vi "SS_acquire_data.vi"(0 "Type":refnum<k20>, 1 "idx":i32, 5 "SweptSines (in)":T3={"Log-Channel_select"=[FALSE, FALSE, FALSE, FALSE, FALSE, FALSE], "JSON Header"="", "SS-Params-Array"=[], "input_frequency_definitions"={"Amp"=0.0, "Ts"=0.0, "num_periodsMT"=[], "freqs_Hz"=[], "numAve_s"=[], "Nsamp_total"=[], "Nsettle_s"=[], "Ncollect_s"=[]}, "DAC-ADC primary 2"=0, "Channel-Names"=[], "num_chan"=0, "num-freqs"=0, "Input File (json)"=path "Z:/mpc-journal/sysID/FRF_data/x-axis_sines_info.json"} {"DAC-ADC primary 2" items=["DAC0/ADC0", "DAC1/ADC1", "DAC2/ADC2", "DAC3/ADC3", ""]}, 11 "error in":errorcluster, 12 "Signal Amplitude (V)":dbl=1.0) -> (4 "FPGA Interface out":T6, 6 "SweptSines (out)":T3={"Log-Channel_select"=[FALSE, FALSE, FALSE, FALSE, FALSE, FALSE], "JSON Header"="", "SS-Params-Array"=[], "input_frequency_definitions"={"Amp"=0.0, "Ts"=0.0, "num_periodsMT"=[], "freqs_Hz"=[], "numAve_s"=[], "Nsamp_total"=[], "Nsettle_s"=[], "Ncollect_s"=[]}, "DAC-ADC primary 2"=0, "Channel-Names"=[], "num_chan"=0, "num-freqs"=0, "Input File (json)"=path "Z:/mpc-journal/sysID/FRF_data/x-axis_sines_info.json"} {"DAC-ADC primary 2" items=["DAC0/ADC0", "DAC1/ADC1", "DAC2/ADC2", "DAC3/ADC3", ""]}, 10 "experiment-data":T1, 15 "error IO":errorcluster)   [LabVIEW 2017]
uses:
  controls/SS_fpga_sysID_REFTYPE.ctl
  controls/SS_SweptSines.ctl
  controls/SS_sin_params.ctl
  controls/SS_input_data_json.ctl
  controls/SS_experimental-data.ctl
  controls/SS_FourierData.ctl
  fpga_interface_lib/fpga_interface_types/fpga-swept-sines-dynamic-ref.ctl
  <vilib>/Utility/error.llb/DialogType.ctl
  <vilib>/Utility/error.llb/Error Cluster From Error Code.vi
  <vilib>/rvi/errors/niLvFpgaAdjustHostInterfaceError.vi
  fpga_interface_lib/acquire_FXP_16-5_FIFO_1.vi
  <vilib>/rvi/interface/nirviReadWriteControl/nirviReadWriteControl.xnode
  c-src/sweptSines_lib/libsweptsines.dll
  fpga_interface_lib/fpga_interface.lvlib
  <vilib>/rvi/interface/Simulation/niFpgaSimulationCallBeginRW.vi
  NiFpgaLv.dll
panel:
  out "Type out":refnum<k20>
  in  "experiment-data--":T1
  in  "DDS_params":T7={"Accumulator Increment"=100000, "Phase Shift"=0, "Signal Amplitude (x 2^15)"=32768}
  out "iter":i32
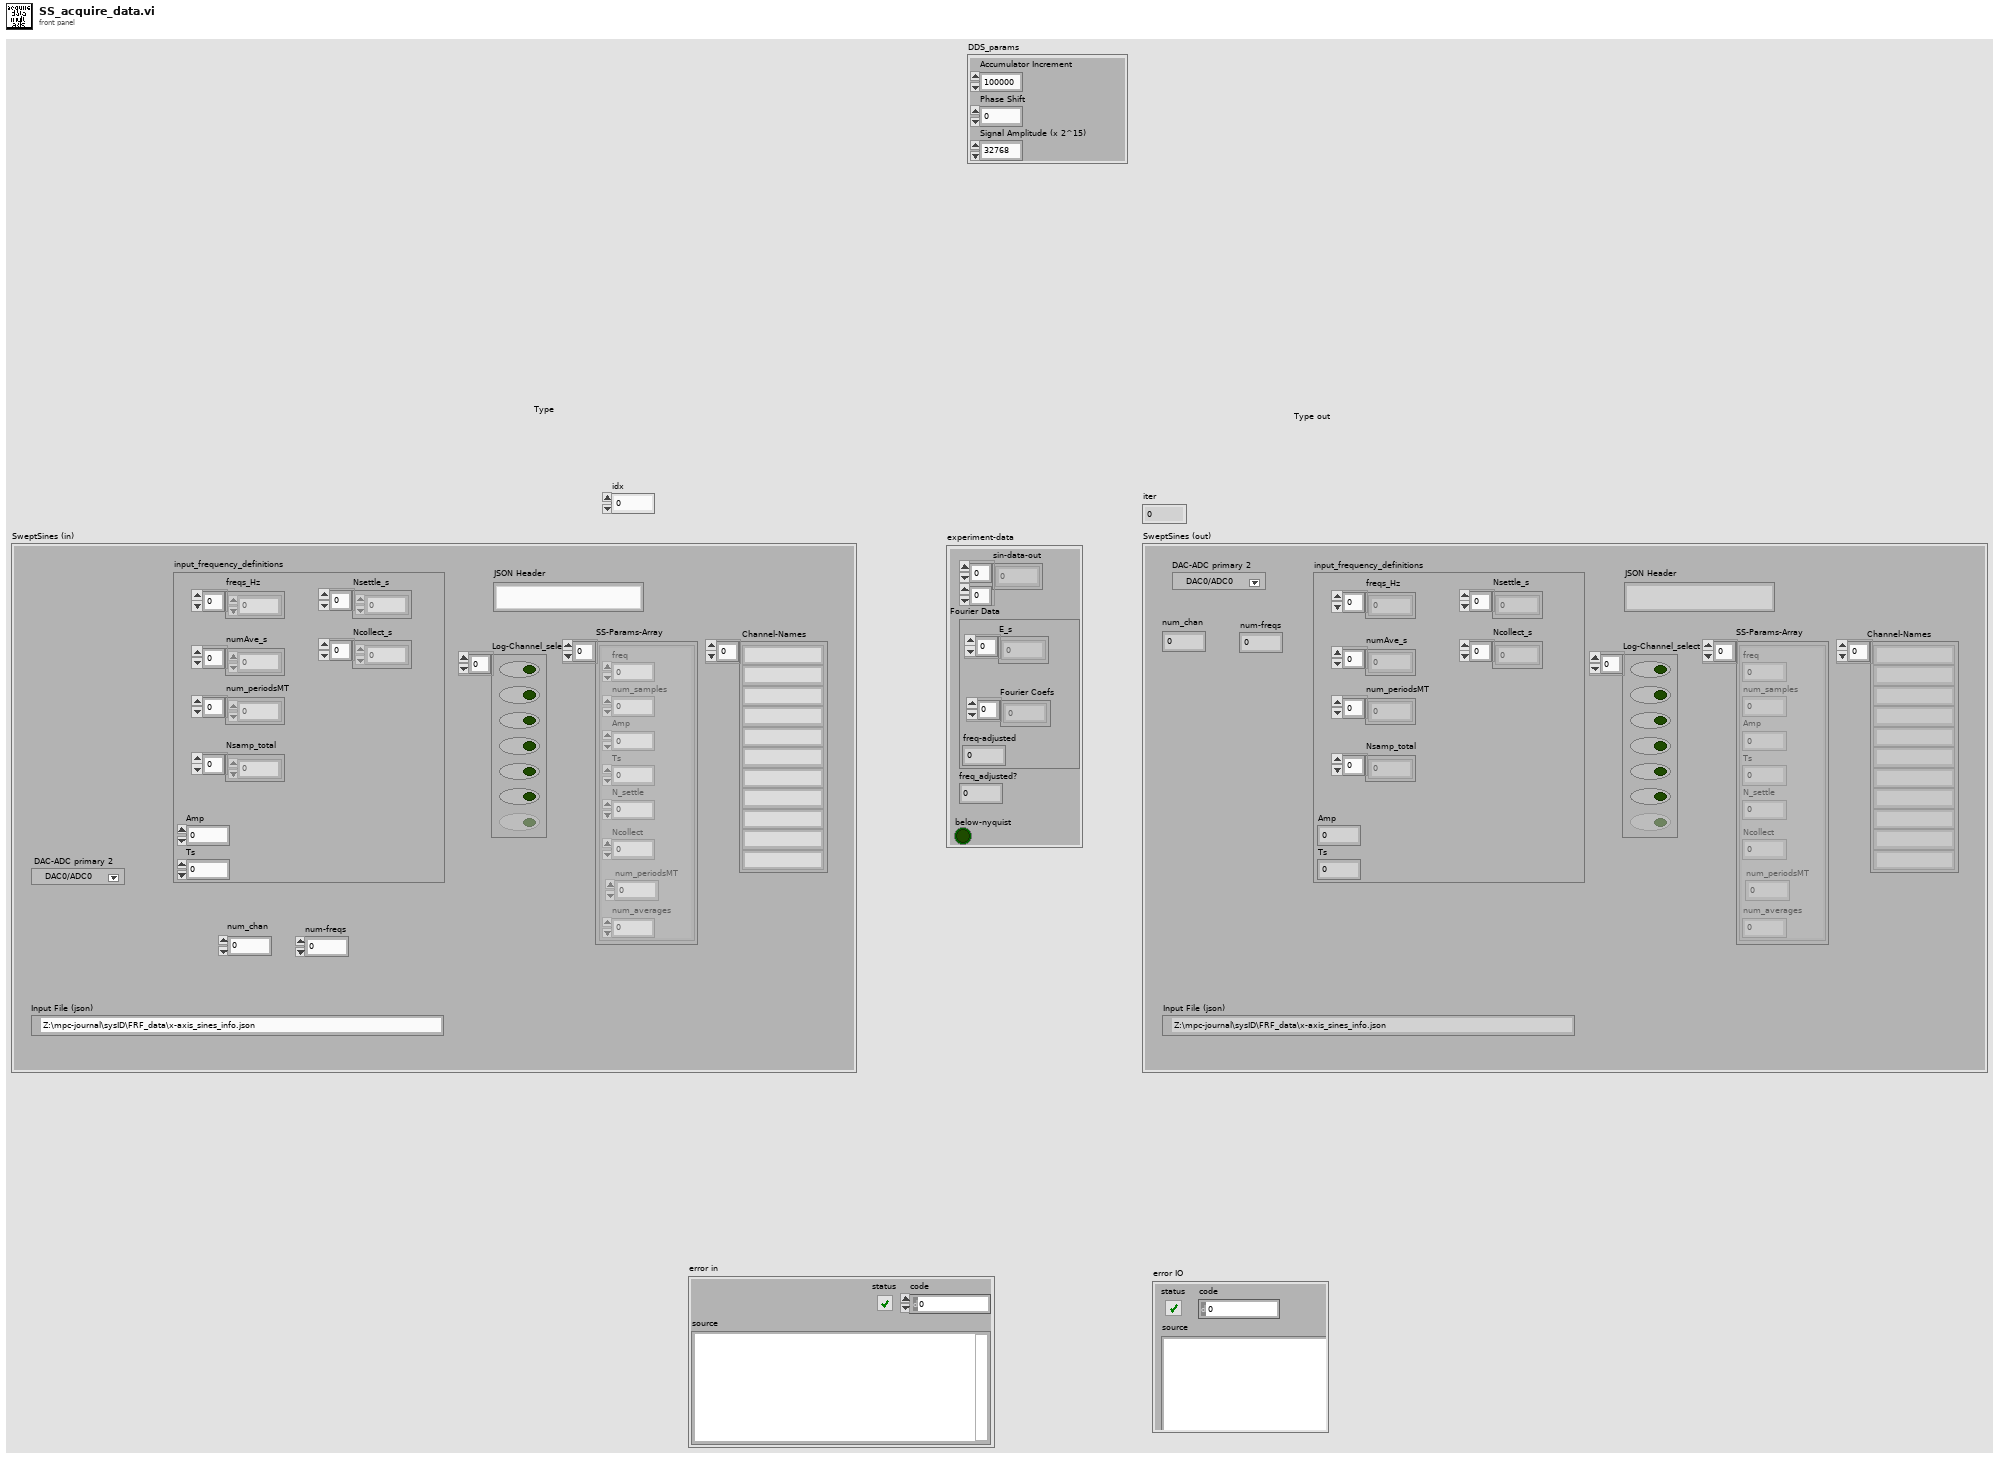
[diagram p1: front panel]
types:
  T1 = typedef "SS_experimental-data.ctl" = cluster{"sin-data-out":dbl[][], "Fourier Data":T2, "freq_adjusted?":dbl, "below-nyquist":bool}
  T2 = typedef "SS_FourierData.ctl" = cluster{"E_s":dbl[], "Fourier Coefs":cdb[], "freq-adjusted":dbl}
  T3 = typedef "SS_SweptSines.ctl" = cluster{"Log-Channel_select":bool[], "JSON Header":string, "SS-Params-Array":T4[], "input_frequency_definitions":T5, "DAC-ADC primary 2":i16, "Channel-Names":string[], "num_chan":i32, "num-freqs":i32, "Input File (json)":path}
  T4 = typedef "SS_sin_params.ctl" = cluster{"freq":dbl, "num_samples":i32, "Amp":dbl, "Ts":dbl, "N_settle":u32, "Ncollect":i32, "num_periodsMT":i32, "num_averages":i32}
  T5 = typedef "SS_input_data_json.ctl" = cluster{"Amp":dbl, "Ts":dbl, "num_periodsMT":u32[], "freqs_Hz":dbl[], "numAve_s":i32[], "Nsamp_total":u32[], "Nsettle_s":u32[], "Ncollect_s":u32[]}
  T6 = typedef "SS_fpga_sysID_REFTYPE.ctl" = refnum<k20>
  T7 = cluster{"Accumulator Increment":u32, "Phase Shift":u32, "Signal Amplitude (x 2^15)":u16}
  T8 = typedef "fpga_interface.lvlib/fpga-swept-sines-dynamic-ref.ctl" = refnum<k20>
  T9 = cluster{"unstable-z-traj":bool, "input fifo time-out":bool, "logging fifo timeout":bool, "scanning finished":bool, "unstable-x-traj":bool, "unstable-y-traj":bool, "ABORT":bool, "All Measurements Done":bool, "fpga_finished":bool, "current_scan_finished":bool}
  T10 = typedef "DialogType.ctl" = u16
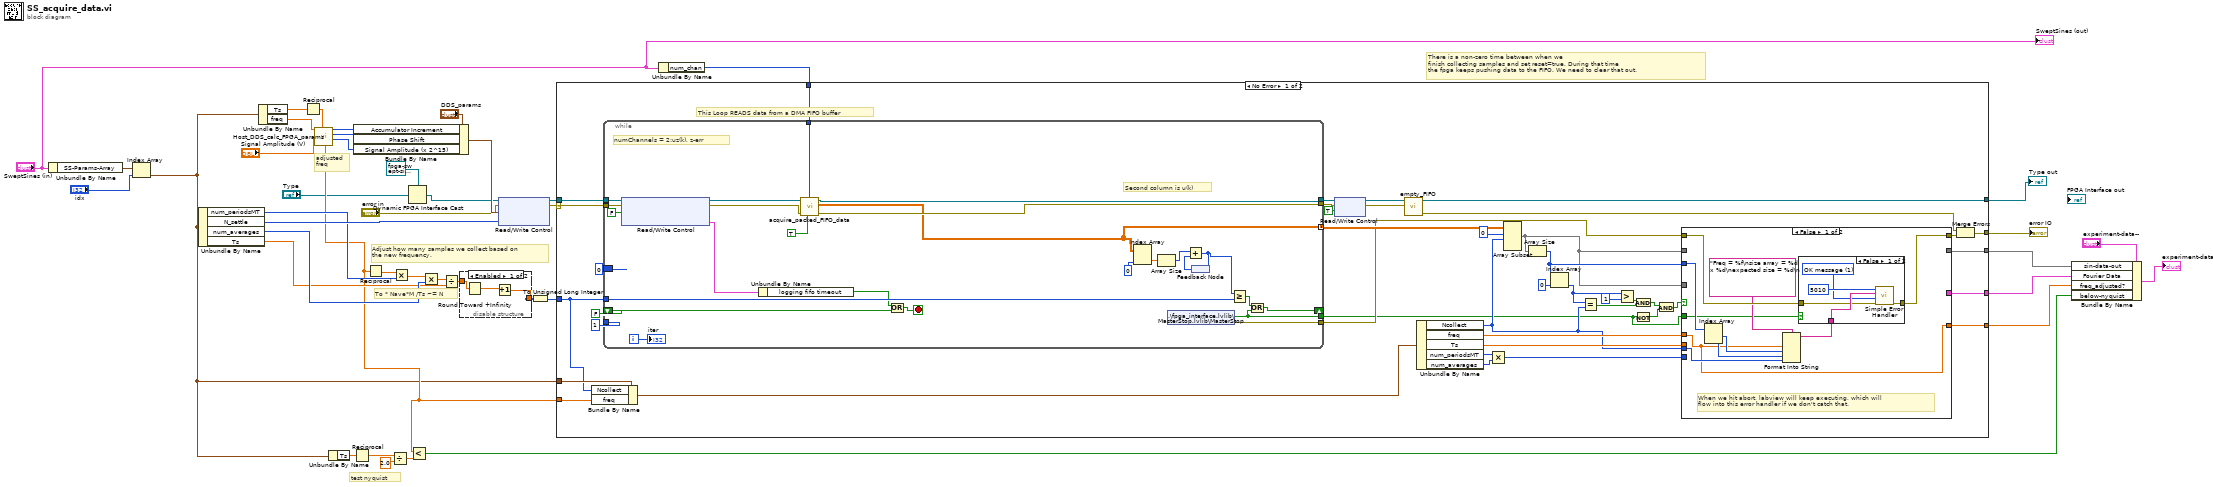
[diagram p0: block diagram]
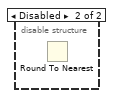
[diagram p2: hidden frame]
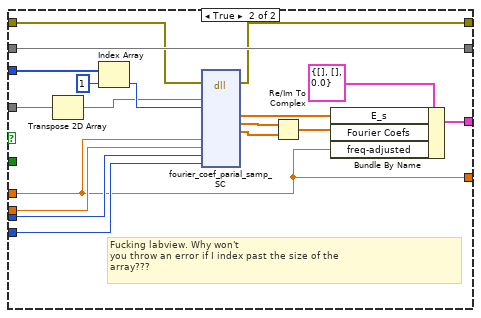
[diagram p4: hidden frame]
diagram:
  # "test nyquist"
  # "There is a non-zero time between when we\nfinish collecting samples and set reset=true. During that time\nthe fpga keeps pushing data to the FIFO. We need to clear that out."
  # "To * Nave*M /Ts ~= N"
  # "adjusted\nfreq"
  # "Adjust how many samples we collect based on\nthe new frequency."
  n1 = Unbundle By Name("SweptSines (in)") -> ("SS-Params-Array"=w15:T4[])
  n2 = Index Array(array=w15, index="idx") -> (element=w13:T4)
  n3 = Unbundle By Name(w13) -> ("num_periodsMT"=w32:i32, "N_settle"=w42:u32, "num_averages"=w28:i32, "Ts"=w25:dbl)
  n4 = Unbundle By Name(w13) -> ("Ts"=w35:dbl, "freq"=w41:dbl)
  n5 = Reciprocal(x=w35) -> (1/x=w36:dbl)
  n6 = call "Host_DDS_calc_FPGA_params.vi"("Loop Rate (Hz)"=w36, "Signal Amplitude (V)"="Signal Amplitude (V)", "DDS Signal Frequency (Hz)"=w41) -> ("AO Amplitude"=w37:u16, "Phase Shift"=w38:u32, "Accumulator Increment"=w39:u32, "freq_adjusted?"=w16:dbl)  [unwired: 5 in]
  n7 = Unbundle By Name(w13) -> ("Ts"=w20:dbl)
  n8 = Reciprocal(x=w20) -> (1/x=w19:dbl)
  n9 = Bundle By Name(cluster="DDS_params", "Accumulator Increment"=w39, "Phase Shift"=w38, "Signal Amplitude (x 2^15)"=w37) -> (w33:T7)
  n10 = Reciprocal(x=w16) -> (1/x=w31:dbl)
  n11 = Divide(x=w19, y=2.0) -> (x/y=w17:dbl)
  n12 = Multiply(x=w31, y=w32) -> (x*y=w27:dbl)
  n13 = Dynamic FPGA Interface Cast(Session In=T8 refnum ("Type"), Type="Type") -> (Session Out=w4:T8)
  n14 = Less?(x=w16, y=w17) -> (x < y?=w5:bool)
  n15 = Multiply(x=w27, y=w28) -> (x*y=w26:dbl)
  n16 = Divide(x=w26, y=w25) -> (x/y=w22:dbl)
  n17 = disable-structure shown="Enabled" {
    disable-tunnel: [w45 _] -> w23
    disable-tunnel: w22 -> [w44 _]
    frame Enabled {
      n18 = Round Toward +Infinity(x=w44) -> (ceil(x): smallest int >= x=w46:dbl)
      n19 = Increment(x=w46) -> (x+1=w45:dbl)
    }
    frame Disabled {
      n20 = Round To Nearest() -> ()  [unwired: 1 in, 1 out]
    }
  }
  n21 = xnode "Read/Write Control"("FPGA VI Reference In"=w4, "error in"="error in", "DDS_params"=w33, "Nsettle"=w42) -> ("FPGA VI Reference Out"=w43:T8, "error out"=w29:errorcluster)
  n22 = To Unsigned Long Integer(number=w23) -> (unsigned 32bit integer=w24:u32)
  n23 = Unbundle By Name("SweptSines (in)") -> ("num_chan"=w11:i32)
  n24 = case shown="No Error" w29 {
    selector: w29 -> [w66 w150]
    tunnel: w43 -> [w85 w149]
    tunnel: w16 -> [w81 w148]
    tunnel: w13 -> [w79 _]
    tunnel: w24 -> [w65 _]
    tunnel: [w77 _] -> w8
    tunnel: [w56 w150] -> w30
    tunnel: [w68 _] -> w7
    tunnel: [w53 w149] -> w1
    tunnel: w11 -> [w52 _]
    tunnel: [w51 w148] -> w6
    frame No Error {
      # "This Loop READS data from a DMA FIFO buffer"
      n25 = Bundle By Name(cluster=w79, "Ncollect"=w65, "freq"=w81) -> (w80:T4)
      n26 = while {
        tunnel: [w128] -> w84
        tunnel: [w127] -> w59
        tunnel: u32 1 -> [_]
        tunnel: w65 -> [w147]
        shift-right: [w143] -> _
        shift-left: FALSE -> [w133]
        tunnel: w85 -> [w139]
        tunnel: w66 -> [w138]
        tunnel: [w131] -> w60
        border: u32 0 -> [_]
        tunnel: [w126] -> w82 mode=concatenating
        tunnel: [w132] -> w47
        tunnel: w52 -> [w129]
        i -> [w136]
        stop <- w135 stop-if-true
        # "numChannels = 2:uz(k), z-err"
        # "Second column is u(k)"
        n27 = xnode "Read/Write Control"("FPGA VI Reference In"=w139, "error in"=w138, "reset"=FALSE) -> ("FPGA VI Reference Out"=w124:T8, "error out"=w130:errorcluster, "boolean  indicators"=w123:T9)
        n28 = Unbundle By Name(w123) -> ("logging fifo timeout"=w134:bool)
        n29 = call-poly "acquire_packed_FIFO_data.vi"("Run once?"=TRUE, "numChannels"=w129, "error in"=w130, "FPGA Interface"=w124) -> ("error out"=w128:errorcluster, "2D Data Out"=w126:dbl[][], "FPGA Interface (out)"=w127:T8)  [unwired: 3 in, 2 out]
        n30 = Or(x=w134, y=w133) -> (x .or. y?=w135:bool)
        n31 = Index Array(array=w126, index (col)=0) -> (element=w141:dbl[])  [unwired: 1 in]
        n32 = Array Size(array=w141) -> (size(s)=w144:i32)
        n33 = shared-variable ".\\fpga_interface.lvlib\\MasterStop.lvlib\\MasterStop"() -> (w132:bool, error out=w131:errorcluster)  [unwired: 1 in]
        n34 = feedback #1() -> (w146:u32)
        n35 = Add(x=w144, y=w146) -> (x+y=w140:u32)
        n36 = feedback-in #1(w140) -> ()
        n37 = Greater Or Equal?(x=w140, y=w147) -> (x >= y?=w142:bool)
        n38 = Or(x=w142, y=w132) -> (x .or. y?=w143:bool)
        "iter" <- w136
      }
      n39 = xnode "Read/Write Control"("FPGA VI Reference In"=w59, "error in"=w84, "reset"=TRUE) -> ("FPGA VI Reference Out"=w58:T8, "error out"=w57:errorcluster)
      n40 = call "empty_FIFO.vi"("error in"=w57, "FPGA Interface"=w58) -> ("error out"=w54:errorcluster, "FPGA Interface out"=w53:T8)  [unwired: 7 in, 1 out]
      n41 = Unbundle By Name(w80) -> ("Ncollect"=w64:i32, "freq"=w76:dbl, "Ts"=w69:dbl, "num_periodsMT"=w63:i32, "num_averages"=w62:i32)
      n42 = Multiply(x=w63, y=w62) -> (x*y=w61:i32)
      n43 = Array Subset(array=w82, index (row)=0 ("index"), length (row)=w64) -> (w67:dbl[][])  [unwired: 2 in]
      n44 = Array Size(array=w67) -> (size(s)=w75:i32[])
      n45 = Index Array(array=w75, index=0) -> (element=w71:i32)
      n46 = Equal?(x=w71, y=w64) -> (x = y?=w73:bool)
      n47 = Greater?(x=w71, y=1) -> (0:w72:bool)
      n48 = And(x=w72, y=w73) -> (x .and. y?=w50:bool)
      n49 = Not(x=w47) -> (.not. x?=w48:bool)
      n50 = And(x=w50, y=w48) -> (x .and. y?=w49:bool)
      n51 = case shown="False" w49 {
        tunnel: w75 -> [w96 w121]
        tunnel: w67 -> [_ w118]
        tunnel: [_ w108] -> w77
        tunnel: w76 -> [w89 w105]
        tunnel: w64 -> [w93 w114]
        tunnel: [w97 w111] -> w55
        tunnel: w60 -> [w98 w112]
        tunnel: w69 -> [_ w115]
        tunnel: w47 -> [w90 _]
        tunnel: [_ w113] -> w68
        tunnel: w67 -> [_ w113]
        tunnel: w61 -> [_ w110]
        tunnel: [w89 w105] -> w51
        frame False {
          # "When we hit abort, labview will keep executing, which will\nflow into this error handler if we don't catch that."
          n52 = Index Array(array=w96) -> (element #1=w95:i32, element #2=w94:i32)  [unwired: 2 in]
          n53 = Format Into String(format string="Freq = %f\nsize array = %d x %d\nexpected size = %d\n ", w89, w95, w94, w93) -> (resulting string=w92:string)  [unwired: 2 in, 1 out]
          n54 = case shown="False" w90 {
            tunnel: w98 -> [w100 w104]
            tunnel: [w103 w104] -> w97
            tunnel: w92 -> [w101 _]
            frame False {
              w99 = T10 1 items=["no dialog", "OK message", "continue or stop message", "OK message + warnings", "continue/stop + warnings"] ("type of dialog (OK msg:1)")
              n55 = call <vilib>:"Simple Error Handler.vi"("error code (no error:0)"=5010, "error source (\" \")"=w101, "type of dialog (OK msg:1)"=w99, "error in (no error)"=w100) -> ("error out"=w103:errorcluster)  [unwired: 1 in, 4 out]
            }
            frame True {
            }
          }
        }
        frame True {
          # "Fucking labview. Why won't\nyou throw an error if I index past the size of the\narray???"
          n56 = Transpose 2D Array(2D array=w118) -> (transposed array=w119:dbl[][])
          n57 = Index Array(array=w121, index=1) -> (element=w122:i32)
          n58 = dll-call lib="C:/Users/arnold/Documents/afm-cs/c-src/sweptSines_lib/libsweptsines.dll" fn="fourier_coef_parial_samp_SC"(error in=w112, "y"=w119, "numChan"=w122, "freq"=w105, "Ts"=w115, "N"=w114, "M"=w110) -> (error out=w111:errorcluster, "E_s"=w107:dbl[], "Yc"=w116:dbl[], "Ys"=w117:dbl[])  [unwired: 12 in, 1 out]
          n59 = Re/Im To Complex(1:w117, 2:w116) -> (0:w106:cdb[])
          n60 = Bundle By Name(cluster=T2 {"E_s"=[], "Fourier Coefs"=[], "freq-adjusted"=0.0} ("Fourier Data 2"), "E_s"=w107, "Fourier Coefs"=w106, "freq-adjusted"=w105) -> (w108:T2)
        }
      }
      n61 = Merge Errors(w54, w55) -> (w56:errorcluster)
    }
    frame Error {
    }
  }
  "error IO" <- w30
  "Type out" <- w1
  n62 = Bundle By Name(cluster="experiment-data--", "sin-data-out"=w7, "Fourier Data"=w8, "freq_adjusted?"=w6, "below-nyquist"=w5) -> (→"experiment-data":T1)
  "SweptSines (out)" <- "SweptSines (in)"
